vi "CANOpen_SDO_FIFO.vi"(7 "nodes":i32, 8 "error in":errorcluster, 11 "Parent":string) -> (0 "error out":errorcluster, 3 "SDO queues":T1)   [LabVIEW 2021, in "CANOpen Addon Engine.lvlib"]
uses:
  CANOpen Addon Engine.lvlib
  CanOpen_SDO queue ref.ctl
  SDO queue.ctl
  Shared/CANOpen_SDO Settings.ctl
  Shared/CANOpen Addon Shared.lvlib
panel:
  # "LSB"
  # "MSB"
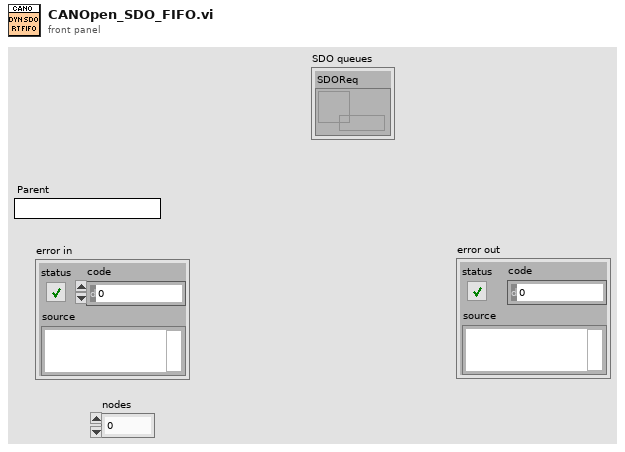
[diagram p1: front panel]
types:
  T1 = typedef "CANOpen Addon Engine.lvlib/CanOpen_SDO queue ref.ctl" = cluster{"SDOReq":refnum<queue>}
  T2 = typedef "CANOpen Addon Engine.lvlib/SDO queue.ctl" = cluster{"element":T3, "Node ID":u8}
  T3 = typedef "CANOpen Addon Shared.lvlib/CANOpen_SDO Settings.ctl" = cluster{"Object Index":u16, "Sub-Index (0)":u8, "Block Data":u8[], "Name":string}
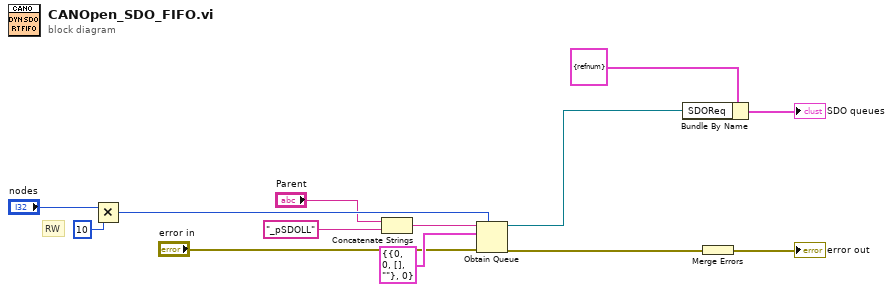
[diagram p0: block diagram]
diagram:
  # "RW"
  n1 = Multiply(x="nodes", y=10) -> (x*y=w3:i32)
  n2 = Concatenate Strings("Parent", "_pSDOLL" ("name (unnamed)")) -> (w12:string)
  n3 = Obtain Queue(max queue size (-1, unlimited)=w3, name (unnamed)=w12, element data type=T2 {"element"={"Object Index"=0, "Sub-Index (0)"=0, "Block Data"=[], "Name"=""}, "Node ID"=0}, error in (no error)="error in") -> (queue out=w6:refnum<queue>, error out=w10:errorcluster)  [unwired: 1 in, 1 out]
  n4 = Bundle By Name(cluster=T1 {"SDOReq"=refnum} ("Queue ref"), "SDOReq"=w6) -> (→"SDO queues":T1)
  n5 = Merge Errors(w10) -> (→"error out":errorcluster)
